vi "Periodic Tasks.vi"(8 "error in":errorcluster) -> ()   [LabVIEW 2013]
doc: "This VI runs in parallel to other tasks. It can contain as many user-defined periodic loops as you need. These can carry out PID or other sorts of timed response."
uses:
  <vilib>/Rock Robotics/SystemInterfaces/DIO/FPGA_DIOChannel.ctl
  <vilib>/Rock Robotics/SystemInterfaces/DIO/FPGA_DIORelayChannel.ctl
  <vilib>/Rock Robotics/WPI/Relay/WPI_RelayValue.ctl
  <vilib>/Rock Robotics/SystemInterfaces/Utilities/FPGA_UtilitiesLED Source.ctl
  <vilib>/Rock Robotics/SystemInterfaces/Utilities/FPGA_UtilitiesLED State.ctl
  Robot Global Data.vi
  <vilib>/Rock Robotics/WPI/Joystick/WPI_JoystickGetSetRefNum.vi
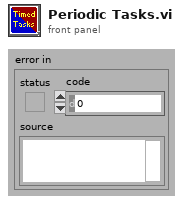
[diagram p1: front panel]
types:
  T1 = typedef "FPGA_DIORelayChannel.ctl" = enum8{"Relay 1", "Relay 2", "Relay 3", "Relay 4", "Relay 5", "Relay 6", "Relay 7", "Relay 8", "Invalid"}
  T2 = typedef "FPGA_DIOChannel.ctl" = enum8{"DIO 1", "DIO 2", "DIO 3", "DIO 4", "DIO 5", "DIO 6", "DIO 7", "DIO 8", "DIO 9", "DIO 10", "DIO 11", "DIO 12", "DIO 13", "DIO 14", "Invalid"}
  T3 = typedef "FPGA_UtilitiesLED State.ctl" = enum16{"Off", "On", "Toggle"}
  T4 = typedef "FPGA_UtilitiesLED Source.ctl" = enum16{"User LED", "FPGA LED"}
  T5 = typedef "WPI_CompressorDevRef.ctl" = cluster{"DevStatus":errorcluster, "DigitalInputDevRef":T6, "RelayDevRef":T8}
  T6 = typedef "WPI_DigitalInputDevRef.ctl" = cluster{"DevStatus":errorcluster, "DIO Channel":T2, "Digital Module":T7}
  T7 = typedef "FPGA_TypedefDigitalModule.ctl" = enum16{"Digital Module 1", "Digital Module 2"}
  T8 = typedef "WPI_RelayDevRef.ctl" = cluster{"DevStatus":errorcluster, "Relay Channel":T1, "Digital Module":T7, "Relay Direction":T9}
  T9 = typedef "WPI_RelayDirection.ctl" = enum16{"Both directions", "Forward only", "Reverse only"}
  T10 = typedef "WPI_JoystickDevRef.ctl" = cluster{"Device":T11}
  T11 = typedef "WPI_JoystickDeviceEnum.ctl" = enum16{"USB 1", "USB 2", "USB 3", "USB 4", "Kinect 1", "Kinect 2"}
  T12 = cluster{"JoystickDevRef":T10, "DigitalInputDevRef":T6}
  T13 = typedef "WPI_RelayValue.ctl" = enum16{"Off", "On", "Forward", "Reverse"}
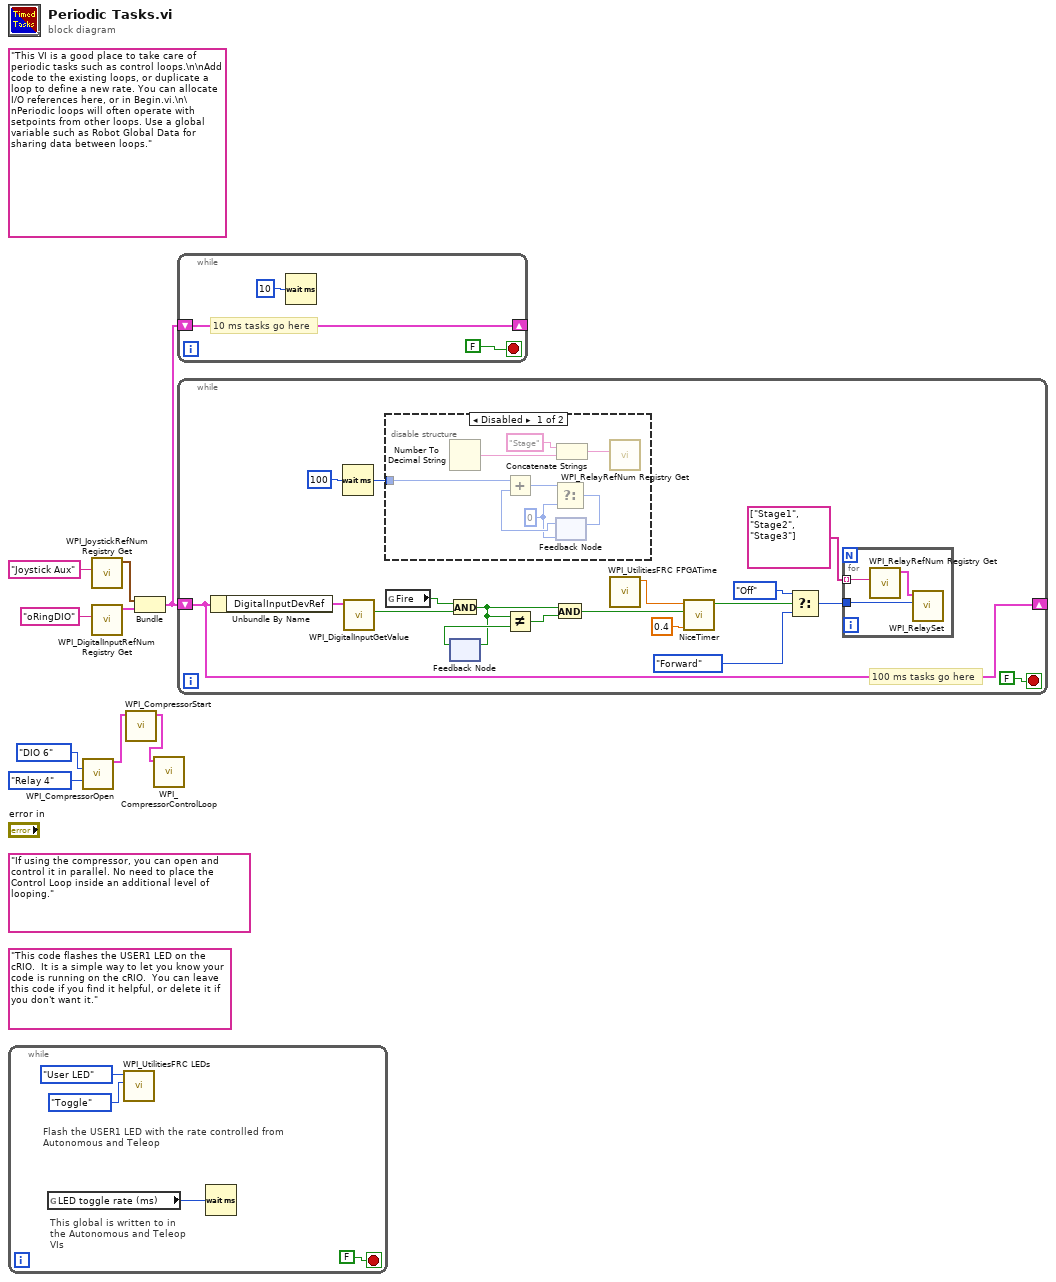
[diagram p0: block diagram]
diagram:
  (unwired) "If using the compressor, you can open and control it in parallel. No need to place the Control Loop inside an additional level of looping."
  (unwired) "This code flashes the USER1 LED on the cRIO.  It is a simple way to let you know your code is running on the cRIO.  You can leave this code if you find it helpful, or delete it if you don't want it."
  (unwired) "This VI is a good place to take care of periodic tasks such as control loops.\n\nAdd code to the existing loops, or duplicate a loop to define a new rate. You can allocate I/O references here, or in Begin.vi.\n\nPeriodic loops will often operate with setpoints from other loops. Use a global variable such as Robot Global Data for sharing data between loops."
  n1 = while {
    stop <- FALSE stop-if-true
    # "This global is written to in the Autonomous and Teleop VIs"
    # "Flash the USER1 LED with the rate controlled from Autonomous and Teleop"
    n2 = global read "Robot Global Data.vi" "LED toggle rate (ms)"() -> (w10:u32)
    n3 = call <vilib>:"WPI_UtilitiesFRC LEDs.vi"("State"=FPGA_UtilitiesLED_State."Toggle", "LED Type"=FPGA_UtilitiesLED_Source."User LED") -> ()  [unwired: 1 in, 9 out]
    n4 = Wait (ms)(milliseconds to wait=w10) -> ()  [unwired: 1 out]
  }
  n5 = call <vilib>:"WPI_CompressorOpen.vi"("Pressure Switch DIO Channel"=FPGA_DIOChannel."DIO 6", "Relay Channel"=FPGA_DIORelayChannel."Relay 4") -> ("CompressorDevRef"=w4:T5)  [unwired: 3 in, 10 out]
  n6 = call <vilib>:"WPI_JoystickRefNum Registry Get.vi"("refnum name"="Joystick Aux") -> ("JoystickDevRef"=w8:T10)  [unwired: 1 in, 9 out]
  n7 = call <vilib>:"WPI_DigitalInputRefNum Registry Get.vi"("refnum name"="oRingDIO") -> ("DigitalInputDevRef"=w2:T6)  [unwired: 9 in, 1 out]
  n8 = call <vilib>:"WPI_CompressorStart.vi"("CompressorDevRef"=w4) -> ("CompressorDevRef"=w1:T5)  [unwired: 9 in, 1 out]
  n9 = Bundle("JoystickDevRef"=w8, "DigitalInputDevRef"=w2) -> (w7:T12)  [unwired: 1 out]
  n10 = call <vilib>:"WPI_CompressorControlLoop.vi"("CompressorDevRef"=w1) -> ()  [unwired: 11 in]
  n11 = while {
    shift-right: [w14] -> _
    shift-left: w7 -> [w14]
    stop <- FALSE stop-if-true
    # "10 ms tasks go here"
    n12 = Wait (ms)(milliseconds to wait=u32 10) -> ()  [unwired: 1 out]
  }
  n13 = while {
    shift-right: [w27] -> _
    shift-left: w7 -> [w27]
    stop <- FALSE stop-if-true
    # "100 ms tasks go here"
    n14 = Unbundle By Name(w27) -> ("DigitalInputDevRef"=w26:T6)
    n15 = Wait (ms)(milliseconds to wait=u32 100) -> (millisecond timer value=w32:u32)
    n16 = call <vilib>:"WPI_DigitalInputGetValue.vi"("DigitalInputDevRef"=w26) -> ("Value"=w25:bool)  [unwired: 8 in, 2 out]
    n17 = disable-structure shown="Disabled" {
      disable-tunnel: w32 -> [w44 _]
      frame Disabled {
        w41 = 0
        n18 = Number To Decimal String() -> (decimal integer string=w38:string)  [unwired: 2 in]
        n19 = feedback #1(w41) -> (w45:i32)
        n20 = Add(x=w44, y=w45) -> (x+y=w43:u32)
        n21 = Select(t=w43, f=w41) -> (s? t:f=w42:u32)  [unwired: 1 in]
        n22 = feedback-in #1(w42) -> ()
        n23 = Concatenate Strings("Stage", w38) -> (w39:string)
        n24 = call <vilib>:"WPI_RelayRefNum Registry Get.vi"("refnum name"=w39) -> ()  [unwired: 9 in, 2 out]
      }
      frame Enabled {
      }
    }
    n25 = global read "Robot Global Data.vi" "Fire"() -> (w22:bool)
    n26 = And(x=w22, y=w25) -> (x .and. y?=w21:bool)
    n27 = feedback #2() -> (w23:bool)  [unwired: 1 in]
    n28 = feedback-in #2(w21) -> ()
    n29 = Not Equal?(x=w21, y=w23) -> (x != y?=w20:bool)
    n30 = And(x=w21, y=w20) -> (x .and. y?=w17:bool)
    n31 = call <vilib>:"WPI_UtilitiesFRC FPGATime.vi"() -> ("FPGA Time"=w24:dbl)  [unwired: 10 in, 1 out]
    n32 = call "NiceTimer.vi"("Wait Duration"=0.4, "Reset Timer"=w17, "Current time"=w24) -> ("Time's up bubby"=w19:bool)  [unwired: 7 in, 1 out]
    n33 = Select(t=WPI_RelayValue."Off", s=w19, f=WPI_RelayValue."Forward" ("RelayValue")) -> (s? t:f=w29:T13)
    n34 = for {
      tunnel: string[] ["Stage1", "Stage2", "Stage3"] -> [w36] mode=indexing
      tunnel: w29 -> [w35]
      n35 = call <vilib>:"WPI_RelayRefNum Registry Get.vi"("refnum name"=w36) -> ("RelayDevRef"=w37:T8)  [unwired: 9 in, 1 out]
      n36 = call <vilib>:"WPI_RelaySet.vi"("RelayValue"=w35, "RelayDevRef"=w37) -> ()  [unwired: 8 in, 2 out]
    }
  }
